vi "Solve2.vi"(8 "Error In":errorcluster, 11 "object in":refnum<class "2021_9.lvclass">) -> (0 "Error Out":errorcluster, 2 "Result":u64, 3 "object out":refnum<class "2021_9.lvclass">)   [LabVIEW 2020, in "2021_9.lvclass"]
uses:
  2021_9.lvclass
  2021_9.lvclass/2021_9.ctl
panel:
  out "x >= y?":bool[][](array[boolean])
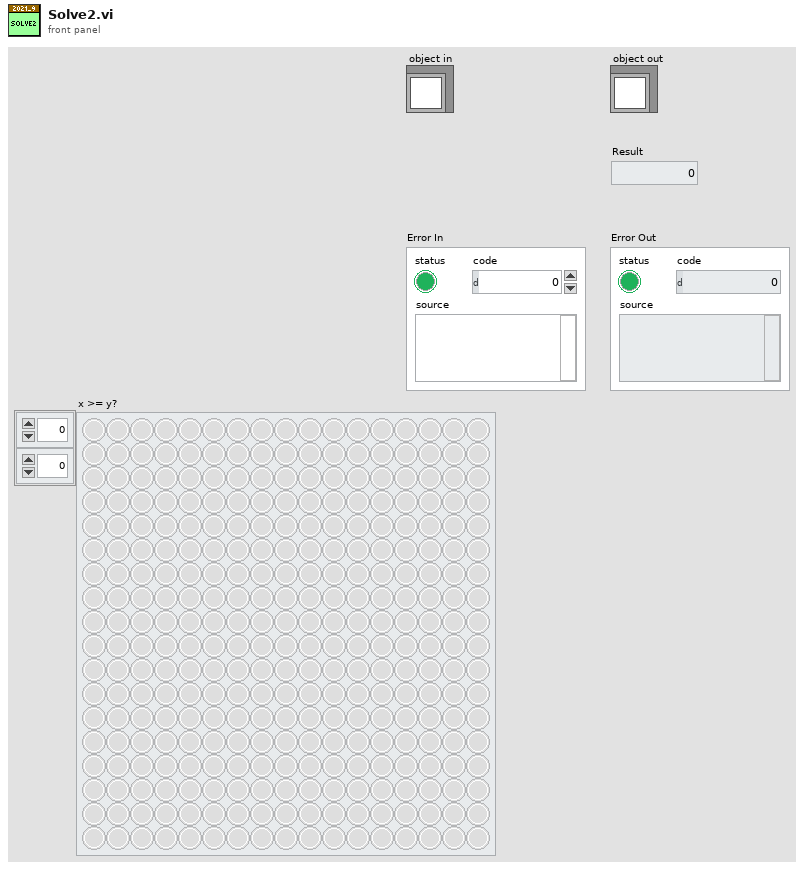
[diagram p1: front panel]
types:
  T1 = cluster{"PixelsFound":cluster{"x":i32, "y":i32}[]}[]
  T2 = cluster{"PixelsFound":cluster{"x":i32, "y":i32}[]}
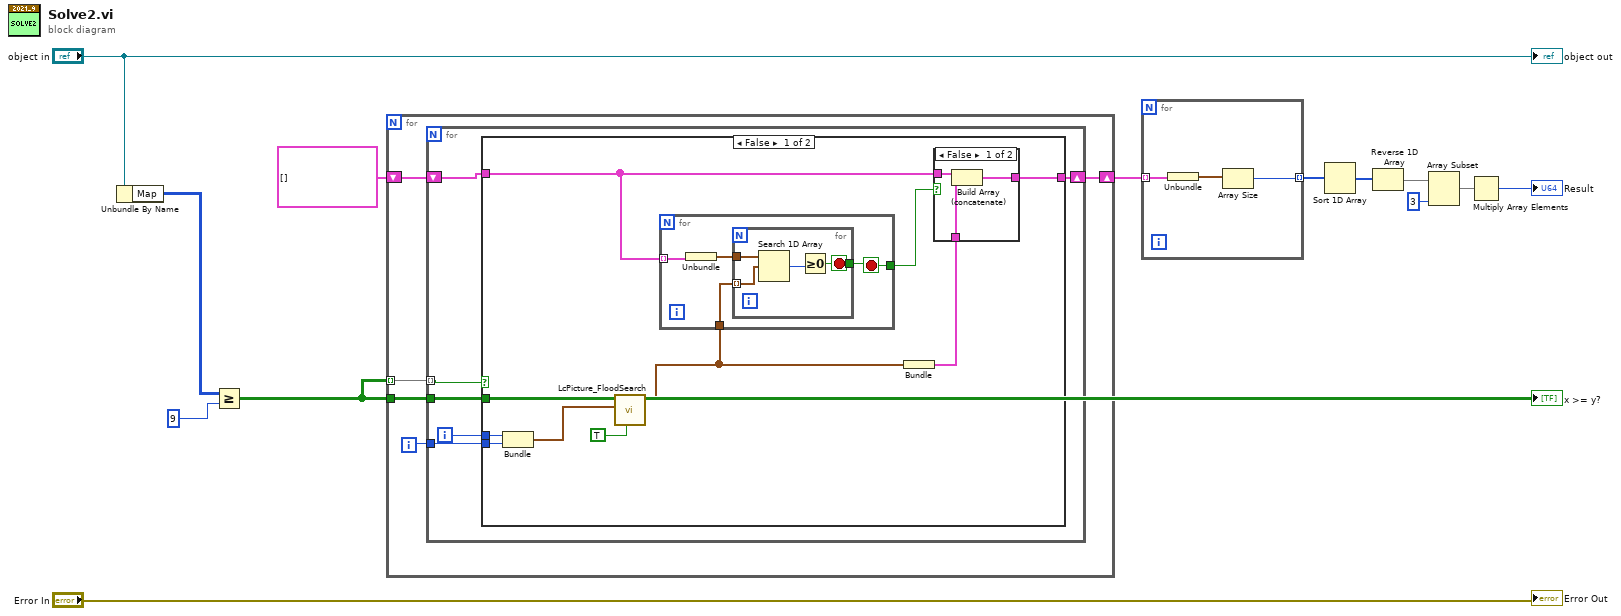
[diagram p0: block diagram]
diagram:
  n1 = Unbundle By Name("object in") -> ("Map"=w3:u8[][])
  n2 = Greater Or Equal?(x=w3, y=u8 9) -> (x >= y?=w4:bool[][])
  "x >= y?" <- w4
  n3 = for {
    tunnel: w4 -> [w18]
    tunnel: w4 -> [w17] mode=indexing
    shift-right: [w14] -> w6
    shift-left: T1 [] -> [w15]
    i -> [w16]
    n4 = for {
      tunnel: w18 -> [w24]
      tunnel: w17 -> [w23] mode=indexing
      tunnel: w16 -> [w21]
      shift-right: [w19] -> w14
      shift-left: w15 -> [w20]
      i -> [w22]
      n5 = case shown="False" w23 {
        tunnel: w24 -> [w33 _]
        tunnel: w22 -> [w32 _]
        tunnel: w21 -> [w31 _]
        tunnel: w20 -> [w27 w47]
        tunnel: [w29 w47] -> w19
        frame False {
          n6 = Bundle(w32, w31) -> (w30:cluster{i32, i32})  [unwired: 1 in]
          n7 = call <userlib>:"LcPicture_FloodSearch.vi"("4 (T) or 8 (F)"=TRUE, "Start Position"=w30, "DataIn"=w33) -> ("PixelsFound"=w26:cluster{"x":i32, "y":i32}[])  [unwired: 5 in, 3 out]
          n8 = for {
            tunnel: w27 -> [w42] mode=indexing
            tunnel: w26 -> [w41]
            tunnel: [w39] -> w25
            stop <- w39 stop-if-true
            n9 = Unbundle(w42) -> ("PixelsFound"=w40:cluster{"x":i32, "y":i32}[])
            n10 = for {
              tunnel: w41 -> [w45] mode=indexing
              tunnel: w40 -> [w46]
              tunnel: [w43] -> w39
              stop <- w43 stop-if-true
              n11 = Search 1D Array(1D array=w46, element=w45) -> (index of element=w44:i32)  [unwired: 1 in]
              n12 = Greater Or Equal To 0?(x=w44) -> (x >= 0?=w43:bool)
            }
          }
          n13 = Bundle("PixelsFound"=w26) -> (w28:T2)  [unwired: 1 in]
          n14 = case shown="False" w25 {
            tunnel: [w37 w38] -> w29
            tunnel: w28 -> [w36 _]
            tunnel: w27 -> [w35 w38]
            frame False {
              n15 = Build Array (concatenate)(w35, w36) -> (w37:T1)
            }
            frame True {
            }
          }
        }
        frame True {
        }
      }
    }
  }
  n16 = for {
    tunnel: w6 -> [w50] mode=indexing
    tunnel: [w48] -> w7 mode=indexing
    n17 = Unbundle(w50) -> ("PixelsFound"=w49:cluster{"x":i32, "y":i32}[])
    n18 = Array Size(array=w49) -> (size(s)=w48:i32)
  }
  n19 = Sort 1D Array(array=w7) -> (sorted array=w8:i32[])
  n20 = Reverse 1D Array(array=w8) -> (reversed array=w9:i32[])
  n21 = Array Subset(array=w9, length=3) -> (w11:i32[])  [unwired: 1 in]
  n22 = Multiply Array Elements(1:w11) -> (0:→"Result":i32)
  "Error Out" <- "Error In"
  "object out" <- "object in"
